vi "CSVRead.vi"(1 "Update Array":bool, 2 "file path (dialog if empty) 2":path=path "U/UntitledPath (7).txt") -> (0 "all rows 2":dbl[][](array[numeric]))   [LabVIEW 2017]
uses:
  <vilib>/Utility/file.llb/Read Delimited Spreadsheet (DBL).vi
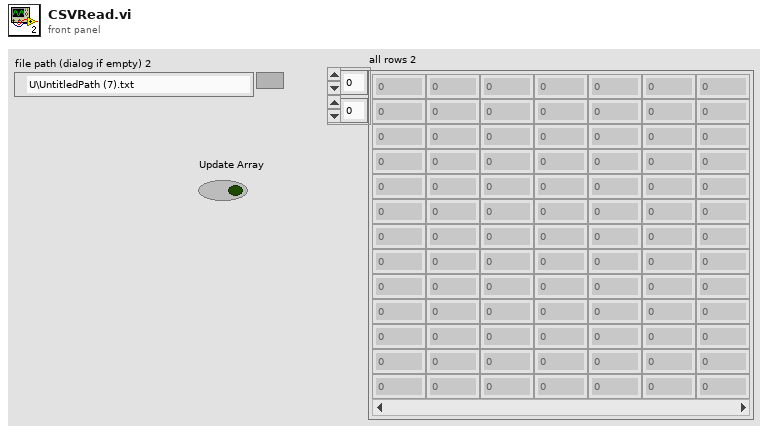
[diagram p1: front panel]
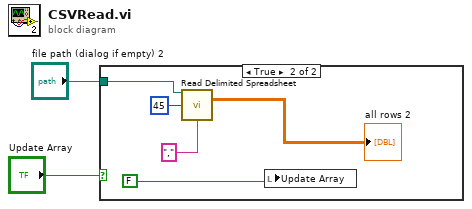
[diagram p0: block diagram]
diagram:
  n1 = case shown="True" "Update Array" {
    tunnel: "file path (dialog if empty) 2" -> [_ w4]
    frame False {
    }
    frame True {
      n2 = call-poly <vilib>:"Read Delimited Spreadsheet.vi"("file path (dialog if empty)"=w4, "start of read offset (chars.:0)"=45, "delimiter (\\t)"="," ("delimiter (\\t)")) -> ("all rows"=→"all rows 2":dbl[][])  [unwired: 7 in, 5 out]
      n3 = local write "Update Array"(FALSE) -> ()
    }
  }
